vi "QueueFinal.vi"() -> ()   [LabVIEW 2021]
panel:
  in  "stop 3":bool
  in  "Button 2":bool
  out "Result":string
  in  "stop 2":bool
  in  "stop":bool
  in  "Button 1":bool
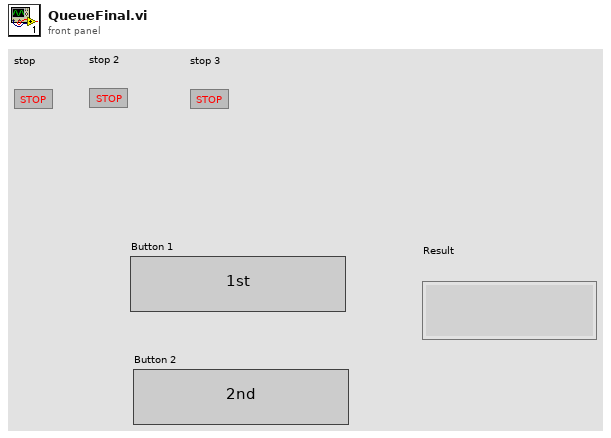
[diagram p1: front panel]
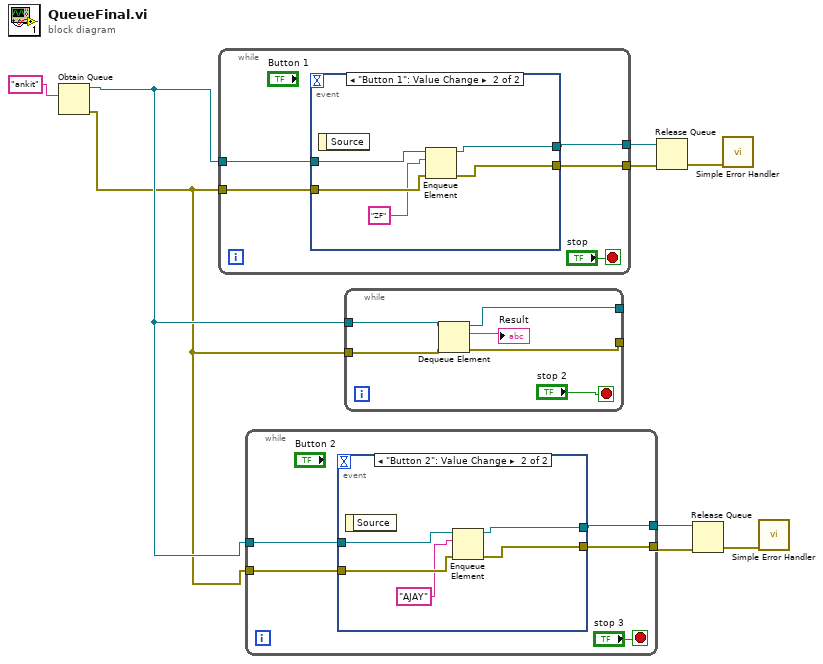
[diagram p0: block diagram]
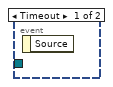
[diagram p2: hidden frame]
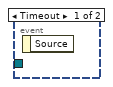
[diagram p3: hidden frame]
diagram:
  n1 = Obtain Queue(element data type="ankit") -> (queue out=w8:refnum<queue>, error out=w7:errorcluster)  [unwired: 4 in, 1 out]
  n2 = while {
    tunnel: w8 -> [w13]
    tunnel: w7 -> [w12]
    tunnel: [w11] -> w5
    tunnel: [w10] -> w6
    stop <- "stop" stop-if-true
    n3 = event shown="[1] \"Button 1\": Value Change" {
      selector: _ -> [_ _]
      dyn-events: _ -> [_ _]
      timeout: _ -> [_ _]
      tunnel: w13 -> [_ w16]
      tunnel: w12 -> [_ w19]
      tunnel: [_ w18] -> w11
      tunnel: [_ w17] -> w10
      event Timeout {
        n4 = event-data() -> ()  [unwired: 1 in, 1 out]
      }
      event "Button 1": Value Change {
        n5 = event-data() -> ()  [unwired: 1 in, 1 out]
        n6 = Enqueue Element(queue=w16, element="ZF", error in (no error)=w19) -> (queue out=w17:refnum<queue>, error out=w18:errorcluster)  [unwired: 1 in, 1 out]
      }
    }
  }
  n7 = while {
    tunnel: w8 -> [w23]
    tunnel: w7 -> [w22]
    tunnel: [w21] -> w1
    tunnel: [w20] -> w2
    stop <- "stop 3" stop-if-true
    n8 = event shown="[1] \"Button 2\": Value Change" {
      selector: _ -> [_ _]
      dyn-events: _ -> [_ _]
      timeout: _ -> [_ _]
      tunnel: w23 -> [_ w26]
      tunnel: w22 -> [_ w29]
      tunnel: [_ w28] -> w21
      tunnel: [_ w27] -> w20
      event Timeout {
        n9 = event-data() -> ()  [unwired: 1 in, 1 out]
      }
      event "Button 2": Value Change {
        n10 = event-data() -> ()  [unwired: 1 in, 1 out]
        n11 = Enqueue Element(queue=w26, element="AJAY", error in (no error)=w29) -> (queue out=w27:refnum<queue>, error out=w28:errorcluster)  [unwired: 1 in, 1 out]
      }
    }
  }
  n12 = while {
    tunnel: w8 -> [w34]
    tunnel: w7 -> [w33]
    tunnel: [w31] -> _
    tunnel: [w30] -> _
    stop <- "stop 2" stop-if-true
    n13 = Dequeue Element(queue=w34, error in (no error)=w33) -> (queue out=w31:refnum<queue>, element=→"Result":string, error out=w30:errorcluster)  [unwired: 1 in, 1 out]
  }
  n14 = Release Queue(queue=w6, error in (no error)=w5) -> (error out=w4:errorcluster)  [unwired: 1 in, 2 out]
  n15 = Release Queue(queue=w2, error in (no error)=w1) -> (error out=w3:errorcluster)  [unwired: 1 in, 2 out]
  n16 = call <vilib>:"Simple Error Handler.vi"("error in (no error)"=w4) -> ()  [unwired: 4 in, 5 out]
  n17 = call <vilib>:"Simple Error Handler.vi"("error in (no error)"=w3) -> ()  [unwired: 4 in, 5 out]
